vi "Periodic Tasks.vi"(8 "error in":errorcluster) -> ()   [LabVIEW 2012]
doc: "This VI runs in parallel to other tasks. It can contain as many user-defined periodic loops as you need. These can carry out PID or other sorts of timed response."
uses:
  ADXL345 I2C Axis.ctl
  <vilib>/Rock Robotics/SystemInterfaces/Utilities/FPGA_UtilitiesLED Source.ctl
  <vilib>/Rock Robotics/SystemInterfaces/Utilities/FPGA_UtilitiesLED State.ctl
  Rec Targeting.vi
  Robot Global Data.vi
  <vilib>/Rock Robotics/WPI/RobotDrive/WPI_RobotDriveGetSetRefNum.vi
  <vilib>/Rock Robotics/WPI/Joystick/WPI_JoystickGetSetRefNum.vi
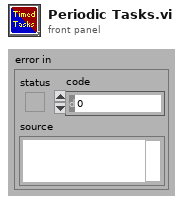
[diagram p1: front panel]
types:
  T1 = typedef "WPI_JoystickDevRef.ctl" = cluster{"Device":T2}
  T2 = typedef "WPI_JoystickDeviceEnum.ctl" = enum16{"USB 1", "USB 2", "USB 3", "USB 4", "Kinect 1", "Kinect 2"}
  T3 = typedef "WPI_RobotDriveDevRef.ctl" = cluster{"DevStatus":errorcluster, "Motors[]":T4[], "Square Inputs":bool, "Max Output":dbl, "Isochronous":bool}
  T4 = typedef "WPI_MotorControlDeviceRef.ctl" = cluster{"DeviceStatus":errorcluster, "Type":enum16{"PWM", "CAN"}, "PWM":cluster{"Digital Module":T5, "PWM Channel":T6, "DeadBand":T7}, "CAN":cluster{"Device Number":u8, "Control Mode":T8, "Semaphore":T9, "Max Vout":dbl}, "Invert":bool, "TransformRef":T10, "InvTransformRef":T10}
  T5 = typedef "FPGA_TypedefDigitalModule.ctl" = enum16{"Digital Module 1", "Digital Module 2"}
  T6 = typedef "FPGA_DIOPWMChannel.ctl" = enum8{"PWM 1", "PWM 2", "PWM 3", "PWM 4", "PWM 5", "PWM 6", "PWM 7", "PWM 8", "PWM 9", "PWM 10", "Invalid"}
  T7 = typedef "WPI_PWMDeadband.ctl" = cluster{"Name":string, "maxPositivePwm":i32, "minPositivePwm":i32, "centerPwm":i32, "maxNegativePwm":i32, "minNegativePwm":i32, "angularRange":u16}
  T8 = typedef "WPI_CANJaguar_ControlMode.ctl" = enum8{"Percent VBus", "Current", "Speed", "Position", "Voltage"}
  T9 = typedef "Semaphore RefNum" = refnum<k1>
  T10 = typedef "WPI_PWMTransform_ConPane.ctl" = refnum<vi>
  T11 = typedef "WPI_I2CDevRef.ctl" = cluster{"DevStatus":errorcluster, "Digital Module":T5, "Device Address":u8}
  T12 = cluster{"JoystickDevRef":T1, "RobotDriveDevRef":T3, "I2CDevRef":T11}
  T13 = typedef "ADXL345 I2C Axis.ctl" = u8
  T14 = typedef "FPGA_UtilitiesLED State.ctl" = enum16{"Off", "On", "Toggle"}
  T15 = typedef "FPGA_UtilitiesLED Source.ctl" = enum16{"User LED", "FPGA LED"}
  T16 = typedef "WPI_CompressorDevRef.ctl" = cluster{"DevStatus":errorcluster, "DigitalInputDevRef":T17, "RelayDevRef":T19}
  T17 = typedef "WPI_DigitalInputDevRef.ctl" = cluster{"DevStatus":errorcluster, "DIO Channel":T18, "Digital Module":T5}
  T18 = typedef "FPGA_DIOChannel.ctl" = enum8{"DIO 1", "DIO 2", "DIO 3", "DIO 4", "DIO 5", "DIO 6", "DIO 7", "DIO 8", "DIO 9", "DIO 10", "DIO 11", "DIO 12", "DIO 13", "DIO 14", "Invalid"}
  T19 = typedef "WPI_RelayDevRef.ctl" = cluster{"DevStatus":errorcluster, "Relay Channel":T20, "Digital Module":T5, "Relay Direction":T21}
  T20 = typedef "FPGA_DIORelayChannel.ctl" = enum8{"Relay 1", "Relay 2", "Relay 3", "Relay 4", "Relay 5", "Relay 6", "Relay 7", "Relay 8", "Invalid"}
  T21 = typedef "WPI_RelayDirection.ctl" = enum16{"Both directions", "Forward only", "Reverse only"}
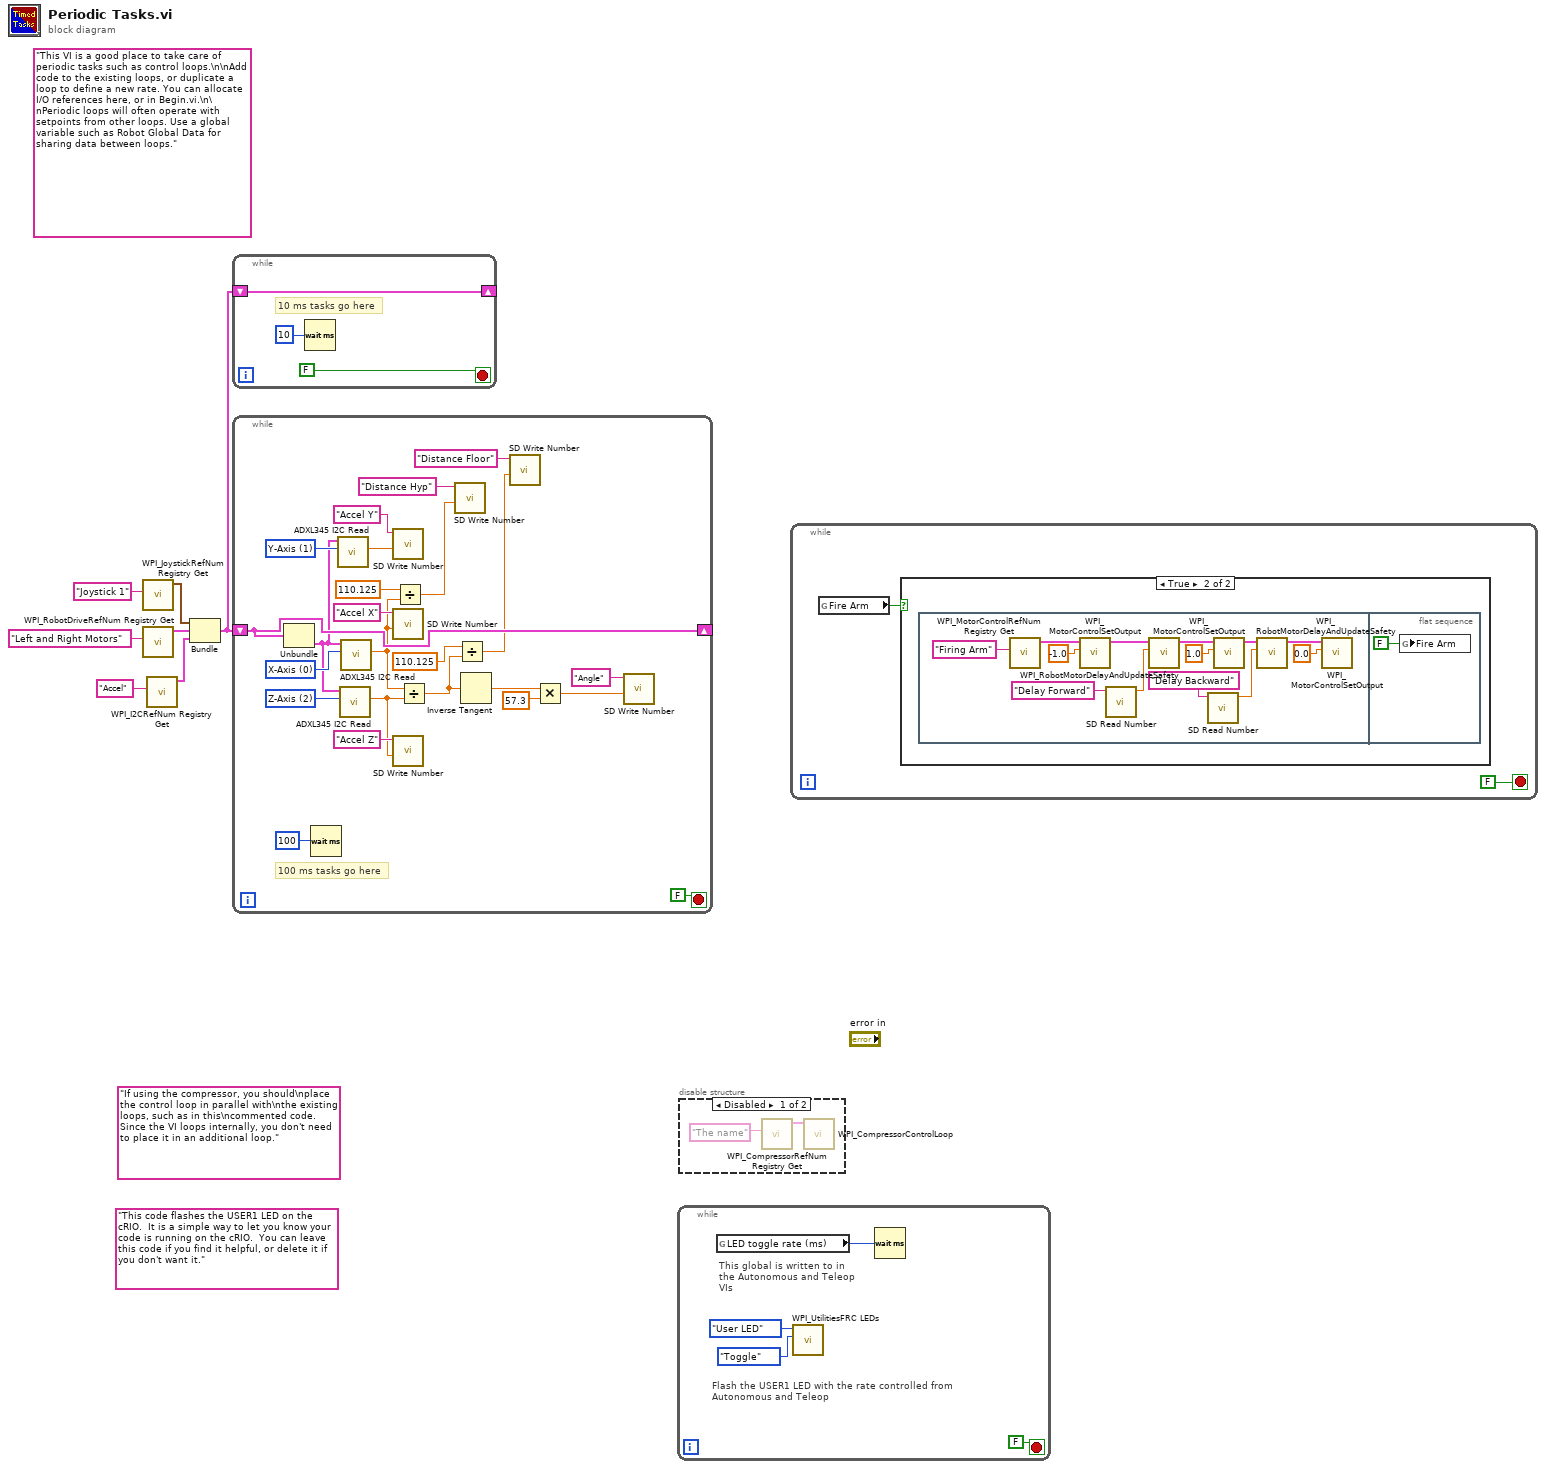
[diagram p0: block diagram]
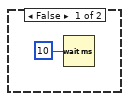
[diagram p2: hidden frame]
diagram:
  (unwired) "If using the compressor, you should\nplace the control loop in parallel with\nthe existing loops, such as in this\ncommented code. Since the VI loops internally, you don't need to place it in an additional loop."
  (unwired) "This code flashes the USER1 LED on the cRIO.  It is a simple way to let you know your code is running on the cRIO.  You can leave this code if you find it helpful, or delete it if you don't want it."
  (unwired) "This VI is a good place to take care of periodic tasks such as control loops.\n\nAdd code to the existing loops, or duplicate a loop to define a new rate. You can allocate I/O references here, or in Begin.vi.\n\nPeriodic loops will often operate with setpoints from other loops. Use a global variable such as Robot Global Data for sharing data between loops."
  n1 = call <vilib>:"WPI_JoystickRefNum Registry Get.vi"("refnum name"="Joystick 1") -> ("JoystickDevRef"=w5:T1)  [unwired: 1 in, 9 out]
  n2 = call <vilib>:"WPI_RobotDriveRefNum Registry Get.vi"("refnum name"="Left and Right Motors") -> ("RobotDriveDevRef"=w4:T3)  [unwired: 1 in, 9 out]
  n3 = call <vilib>:"WPI_I2CRefNum Registry Get.vi"("refnum name"="Accel") -> ("I2CDevRef"=w2:T11)  [unwired: 9 in, 1 out]
  n4 = Bundle("JoystickDevRef"=w5, "RobotDriveDevRef"=w4, "I2CDevRef"=w2) -> (w3:T12)  [unwired: 1 out]
  n5 = while {
    shift-right: [w8] -> _
    shift-left: w3 -> [w8]
    stop <- FALSE stop-if-true
    # "10 ms tasks go here"
    n6 = Wait (ms)(milliseconds to wait=u32 10) -> ()  [unwired: 1 out]
  }
  n7 = while {
    shift-right: [w32] -> _
    shift-left: w3 -> [w32]
    stop <- FALSE stop-if-true
    w29 = T13 1 items=["X-Axis", "Y-Axis", "Z-Axis"] ("Axis")
    w30 = T13 2 items=["X-Axis", "Y-Axis", "Z-Axis"] ("Axis")
    w31 = T13 0 items=["X-Axis", "Y-Axis", "Z-Axis"] ("Axis")
    # "100 ms tasks go here"
    n8 = Unbundle(w32) -> ("I2CDevRef"=w28:T11)  [unwired: 2 out]
    n9 = Wait (ms)(milliseconds to wait=u32 100) -> ()  [unwired: 1 out]
    n10 = call "ADXL345 I2C Read.vi"("Axis"=w29, "I2CDevRef"=w28) -> ("Acceleration"=w23:dbl)  [unwired: 7 in, 2 out]
    n11 = call "ADXL345 I2C Read.vi"("Axis"=w30, "I2CDevRef"=w28) -> ("Acceleration"=w21:dbl)  [unwired: 7 in, 2 out]
    n12 = call "ADXL345 I2C Read.vi"("Axis"=w31, "I2CDevRef"=w28) -> ("Acceleration"=w20:dbl)  [unwired: 7 in, 2 out]
    n13 = call <vilib>:"SD Write Number.vi"("Numeric"=w23, "Name"="Accel Y") -> ()  [unwired: 8 in, 2 out]
    n14 = call <vilib>:"SD Write Number.vi"("Numeric"=w20, "Name"="Accel X") -> ()  [unwired: 8 in, 2 out]
    n15 = call <vilib>:"SD Write Number.vi"("Numeric"=w21, "Name"="Accel Z") -> ()  [unwired: 8 in, 2 out]
    n16 = Divide(x=110.125 ("y"), y=w20) -> (x/y=w18:dbl)
    n17 = Divide(x=w20, y=w21) -> (x/y=w17:dbl)
    n18 = call <vilib>:"SD Write Number.vi"("Numeric"=w18, "Name"="Distance Hyp") -> ()  [unwired: 8 in, 2 out]
    n19 = Divide(x=110.125 ("y"), y=w17) -> (x/y=w14:dbl)
    n20 = Inverse Tangent(1:w17) -> (0:w13:dbl)
    n21 = call <vilib>:"SD Write Number.vi"("Numeric"=w14, "Name"="Distance Floor") -> ()  [unwired: 8 in, 2 out]
    n22 = Multiply(x=w13, y=57.3) -> (x*y=w12:dbl)
    n23 = call <vilib>:"SD Write Number.vi"("Numeric"=w12, "Name"="Angle") -> ()  [unwired: 8 in, 2 out]
  }
  n24 = while {
    stop <- FALSE stop-if-true
    # "This global is written to in the Autonomous and Teleop VIs"
    # "Flash the USER1 LED with the rate controlled from Autonomous and Teleop"
    n25 = global read "Robot Global Data.vi" "LED toggle rate (ms)"() -> (w35:u32)
    n26 = call <vilib>:"WPI_UtilitiesFRC LEDs.vi"("State"=FPGA_UtilitiesLED_State."Toggle", "LED Type"=FPGA_UtilitiesLED_Source."User LED") -> ()  [unwired: 1 in, 9 out]
    n27 = Wait (ms)(milliseconds to wait=w35) -> ()  [unwired: 1 out]
  }
  n28 = disable-structure shown="Disabled" {
    frame Disabled {
      n29 = call <vilib>:"WPI_CompressorRefNum Registry Get.vi"("refnum name"="The name") -> ("CompressorDevRef"=w40:T16)  [unwired: 9 in, 1 out]
      n30 = call <vilib>:"WPI_CompressorControlLoop.vi"("CompressorDevRef"=w40) -> ()  [unwired: 11 in]
    }
    frame Enabled {
    }
  }
  n31 = while {
    stop <- FALSE stop-if-true
    n32 = global read "Rec Targeting.vi" "Fire Arm"() -> (w42:bool)
    n33 = case shown="True" w42 {
      frame False {
        n34 = Wait (ms)(milliseconds to wait=u32 10) -> ()  [unwired: 1 out]
      }
      frame True {
        n35 = flat-sequence {
          frame #0 {
            n36 = call <vilib>:"WPI_MotorControlRefNum Registry Get.vi"("refnum name"="Firing Arm") -> ("MotorControlDevRef"=w55:T4)  [unwired: 9 in, 1 out]
            n37 = call <vilib>:"WPI_MotorControlSetOutput.vi"("Output"=-1.0, "MotorControlDevRef"=w55) -> ("MotorControlDevRef"=w53:T4)  [unwired: 7 in, 2 out]
            n38 = call <vilib>:"SD Read Number.vi"("Name"="Delay Forward") -> ("Numeric"=w45:dbl)  [unwired: 8 in, 2 out]
            n39 = call "WPI_RobotMotorDelayAndUpdateSafety.vi"("Delay (s)"=w45, "MotorControlDevRef"=w53) -> ("MotorControlDevRef 2"=w51:T4)  [unwired: 8 in, 1 out]
            n40 = call <vilib>:"SD Read Number.vi"("Name"="Delay Backward") -> ("Numeric"=w44:dbl)  [unwired: 8 in, 2 out]
            n41 = call <vilib>:"WPI_MotorControlSetOutput.vi"("Output"=1.0, "MotorControlDevRef"=w51) -> ("MotorControlDevRef"=w48:T4)  [unwired: 7 in, 2 out]
            n42 = call "WPI_RobotMotorDelayAndUpdateSafety.vi"("Delay (s)"=w44, "MotorControlDevRef"=w48) -> ("MotorControlDevRef 2"=w49:T4)  [unwired: 8 in, 1 out]
            n43 = call <vilib>:"WPI_MotorControlSetOutput.vi"("Output"=0.0, "MotorControlDevRef"=w49) -> ()  [unwired: 7 in, 3 out]
          }
          frame #1 {
            n44 = global write "Rec Targeting.vi" "Fire Arm"(FALSE ("Fire Arm")) -> ()
          }
        }
      }
    }
  }
